vi "SetRegimeBoundaries.vi"(10 "Default regime boundaries":T1=[0, 70, 140, 220, 190, 290], 11 "Last Commanded Boat Regime":T2={"Sailing Regime"=enum."Tack - Bow across wind", "Emergency Regimes"=enum."No Knockdown", "Emergency?"=FALSE}) -> (3 "Altered regime boundaries":T1=[0, 70, 140, 220, 190, 360])   [LabVIEW 2013]
doc: "This VI defines the boundaries of the Sailing Regimes, and does so using a deadband. What that means is that there is 10 degrees (arbitrary at the moment) of space in between two regimes that doesn't cause a regime shift.\n\nExample: If the boat is in Regime 1, and at 70 degrees from the wind the boat is supposed to go into Regime 2 (that's the default), this VI will push the Regime 1/Regime 2 boundary up to 75 degrees. As soon as the boat hits 75 degrees from the wind and goes into Regime 2, this VI pushes that dividing line back to 65 degrees. Thus there are 10 degrees of variability in betwen each regime. The point of this deadband is so that if the boat is commanded to go to, say, 68 degrees, the shifted boundaries will keep the boat in Regime 1 even when there is +/- 5 degree variability on the relative wind or the boat heading. The point of the deadband is to keep the boat from switching regimes too much when it's near an edge. The range of border variability should be little enough that it doesn't affect sail logic (e.g. the sail logic for Regime 1 should work alright at both 70 and 75 degrees .\n\nEric Schneider, Feb. 2014"
uses:
  Data/TypeDefs/Boat Regimes.ctl
  Data/TypeDefs/Sailing Regimes.ctl
  Data/TypeDefs/Emergency Regimes.ctl
  Data/TypeDefs/Regime Boundaries.ctl
panel:
  in  "Dead Zone Range (deg)":i32=5
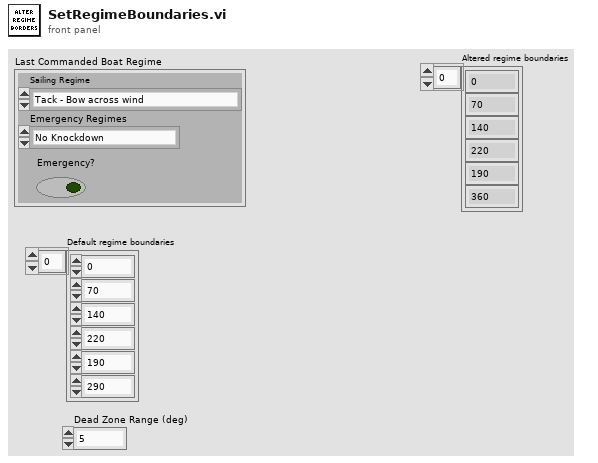
[diagram p1: front panel]
types:
  T1 = typedef "Regime Boundaries.ctl" = i32[]
  T2 = typedef "Boat Regimes.ctl" = cluster{"Sailing Regime":T3, "Emergency Regimes":T4, "Emergency?":bool}
  T3 = typedef "Sailing Regimes.ctl" = enum16{"Tack - Bow across wind", "Upwind - Port Tack", "Turn between Upwind/Reach - Port Tack", "Reach - Port Tack", "Turn between Reach/Run - Port Tack", "Run - Port Tack", "Jibe - Stern across wind", "Run - Starboard Tack", "Turn between Reach/Run - Starboard Tack", "Reach - Starboard Tack", "Turn between Upwind/Reach - Starboard Tack", "Upwind - Starboard Tack"}
  T4 = typedef "Emergency Regimes.ctl" = enum16{"NO EMERGENCY", "No Knockdown", "Obstacle Avoid"}
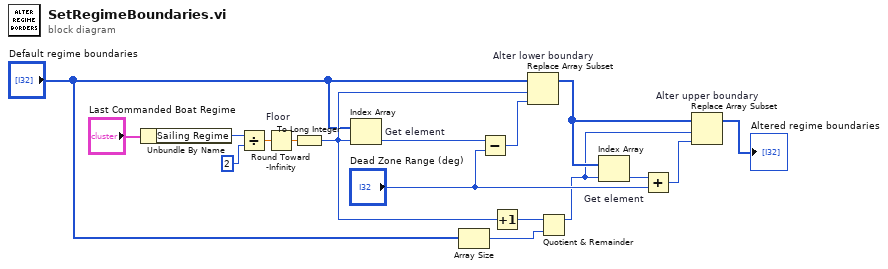
[diagram p0: block diagram]
diagram:
  n1 = Unbundle By Name("Last Commanded Boat Regime") -> ("Sailing Regime"=w16:T3)
  n2 = Divide(x=w16, y=2) -> (x/y=w9:dbl)
  n3 = Round Toward -Infinity "Floor"(1:w9) -> (0:w8:dbl)
  n4 = To Long Integer(number=w8) -> (32bit integer=w7:i32)
  n5 = Index Array "Get element"(array="Default regime boundaries", index=w7) -> (element=w14:i32)
  n6 = Array Size(array="Default regime boundaries") -> (size(s)=w4:i32)
  n7 = Subtract(x=w14, y="Dead Zone Range (deg)") -> (x-y=w6:i32)
  n8 = Increment(x=w7) -> (x+1=w5:i32)
  n9 = Replace Array Subset "Alter lower boundary"(array="Default regime boundaries", new element=w6, index=w7) -> (w10:T1)
  n10 = Quotient & Remainder(x=w5, y=w4) -> (x-y*floor(x/y)=w3:i32)  [unwired: 1 out]
  n11 = Index Array "Get element"(array=w10, index=w3) -> (element=w13:i32)
  n12 = Add(x=w13, y="Dead Zone Range (deg)") -> (x+y=w11:i32)
  n13 = Replace Array Subset "Alter upper boundary"(array=w10, new element=w11, index=w3) -> (→"Altered regime boundaries":T1)
